vi "Init Transition.vi"(7 "VolatusAPI":refnum<class "VolatusAPI.lvclass">, 8 "error in (no error)":refnum<class "MultiErrors.lvclass">, 10 "Transition Config":refnum<class "Transition Config.lvclass">, 11 "State Transition in":refnum<class "State Transition.lvclass">) -> (0 "error out":refnum<class "MultiErrors.lvclass">, 3 "State Transition out":refnum<class "State Transition.lvclass">)   [LabVIEW 2020, in "VolatusSeq.lvlib" / "State Transition.lvclass"]
uses:
  State Transition.lvclass
  Volatus/VolatusAPI/VolatusAPI.lvclass
  VolatusSeqConfig/Transition Config/Transition Config.lvclass
  VolatusSeqConfig/State Transition Config/State Transition Config.lvclass
  VolatusSeqConfig/State Transition Config/State Transition Config.lvclass/State Transition Config.ctl
  State Transition.lvclass/State Transition.ctl
  Volatus/MultiErrors/MultiErrors.lvclass
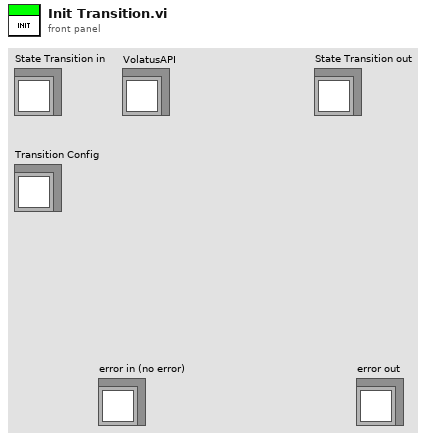
[diagram p1: front panel]
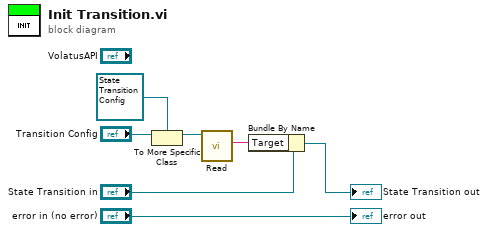
[diagram p0: block diagram]
diagram:
  n1 = To More Specific Class(target class=refnum<class "State Transition Config.lvclass"> refnum ("VolatusSeqConfig.lvlib:State Transition Config.lvclass"), reference="Transition Config") -> (specific class reference=w3:refnum<class "State Transition Config.lvclass">)  [unwired: 1 in, 1 out]
  n2 = call "Read.vi"("State Transition Config in"=w3) -> ("Target State"=w1:string)  [unwired: 10 in]
  n3 = Bundle By Name(cluster="State Transition in", "Target"=w1) -> (→"State Transition out":refnum<class "State Transition.lvclass">)
  "error out" <- "error in (no error)"
